vi "QSM_Push Group to Queue.vi"(8 "error in (no error)":errorcluster, 10 "Group Cmds to Push":T2[](array[typedef]), 11 "QSMRef in":T1) -> (0 "error out":errorcluster, 3 "QSMRef out":T1)   [LabVIEW 2014, in "GUIUpdateQSM.lvlib"]
uses:
  GUIUpdateQSM.lvlib
  Controls/QSM_RunStates.ctl
  Controls/QSM_Reference.ctl
  Controls/QSM_DataType.ctl
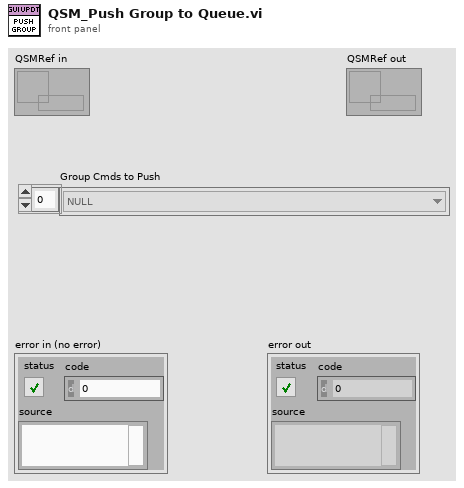
[diagram p1: front panel]
types:
  T1 = typedef "GUIUpdateQSM.lvlib/QSM_Reference.ctl" = refnum<queue>
  T2 = typedef "GUIUpdateQSM.lvlib/QSM_RunStates.ctl" = enum16{"NULL", "Sect01_Initialize-00_GROUP.ENQUEUE", "Sect01_Initialize-01_SetMainToDefault", "Sect01_Initialize-02_Clear Status Strings", "Sect02_UpdateUI-00_Enable Stop_ Disable Start", "Sect02_UpdateUI-01_Enable Start_Disable Stop", "Sect02_UpdateUI-02_Update Status String", "Sect02_UpdateUI-03_Clear XY-Graph", "Sect03-Open ROI  GUI", "Sect03-Close ROI GUI", "Sect99_EXIT-00_Group.Enqueue", "Sect99_EXIT-01_CloseReferences", "Sect99_EXIT-02_StopQSM"}
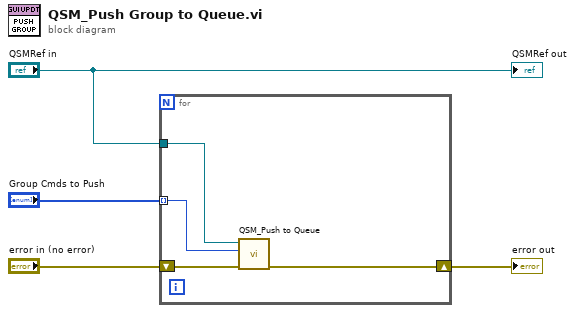
[diagram p0: block diagram]
diagram:
  n1 = for {
    tunnel: "QSMRef in" -> [w5]
    shift-right: [w8] -> w4
    shift-left: "error in (no error)" -> [w7]
    tunnel: "Group Cmds to Push" -> [w6] mode=indexing
    n2 = call "QSM_Push to Queue.vi"("error in (no error)"=w7, "QSM_RunStates"=w6, "QSMRef in"=w5) -> ("error out"=w8:errorcluster)  [unwired: 7 in, 1 out]
  }
  "error out" <- w4
  "QSMRef out" <- "QSMRef in"
